vi "fgt get controllers info.vi"(8 "error in (no error)":errorcluster) -> (0 "error out":errorcluster, 3 "Controllers channels info":T1[](array[typedef]))   [LabVIEW 2016, in "fgt_SDK.lvlib"]
doc: "Retrieve information about session controllers. Controllers are MFCS, Flowboard, Link, IPS and Switchboard."
uses:
  fgt_SDK.lvlib
  TypeDefs/fgt_CONTROLLER_INFO.ctl
  TypeDefs/fgt_INSTRUMENT_TYPE.ctl
  dlls/fgt_SDK_32.dll
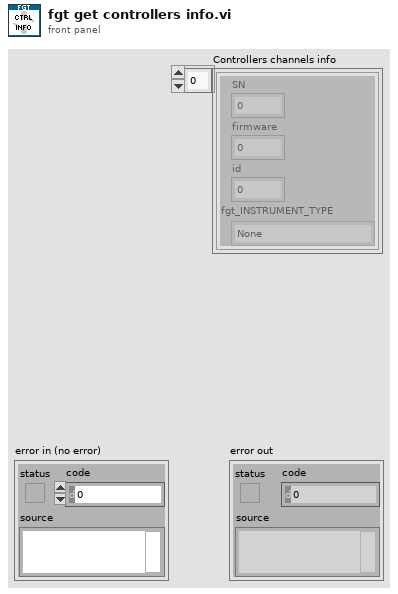
[diagram p1: front panel]
types:
  T1 = typedef "fgt_SDK.lvlib/fgt_CONTROLLER_INFO.ctl" = cluster{"SN":u16, "firmware":u16, "id":u32, "fgt_INSTRUMENT_TYPE":T2}
  T2 = typedef "fgt_SDK.lvlib/fgt_INSTRUMENT_TYPE.ctl" = enum32{"None", "MFCS", "MFCS_EZ", "FRP", "LineUP", "IPS"}
  T3 = typedef "fgt_SDK.lvlib/fgt_STATUS_INFO.ctl" = cluster{"InstrType":T2, "instrSN":u16, "errorCode":u8, "infoCode":u8, "detail":string}
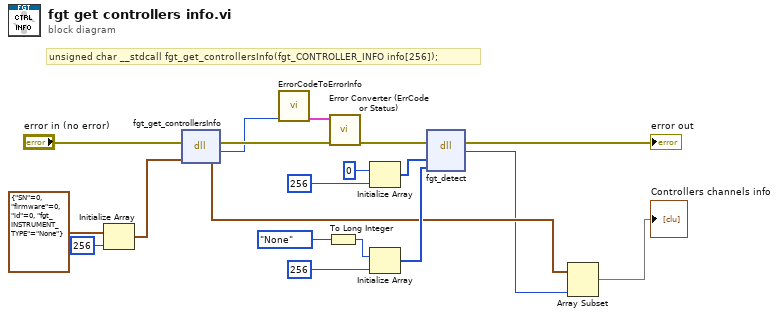
[diagram p0: block diagram]
diagram:
  # "unsigned char __stdcall fgt_get_controllersInfo(fgt_CONTROLLER_INFO info[256]);"
  n1 = Initialize Array(T1 {"SN"=0, "firmware"=0, "id"=0, "fgt_INSTRUMENT_TYPE"=enum."None"} ("fgt_CONTROLLER_INFO"), 256 ("dimension size")) -> (w13:T1[])
  n2 = dll-call lib="C:/projects/SDK/fgt-sdk-labview/dlls/fgt_SDK_*.*" fn="fgt_get_controllersInfo"(error in="error in (no error)", "info"=w13) -> (error out=w18:errorcluster, "return type"=w17:u8, "info"=w3:T1[])  [unwired: 2 in, 1 out]
  n3 = call "ErrorCodeToErrorInfo.vi"("return type"=w17) -> ("StatusInfo"=w16:T3)  [unwired: 10 in]
  n4 = To Long Integer(number=fgt_INSTRUMENT_TYPE."None" ("fgt_INSTRUMENT_TYPE")) -> (32bit integer=w7:i32)
  n5 = call "Error Converter (ErrCode or Status).vi"("error in (no error)"=w18, "StatusInfo"=w16) -> ("error out"=w5:errorcluster)  [unwired: 9 in]
  n6 = Initialize Array(u16 0 ("element"), 256 ("dimension size")) -> (w6:u16[])
  n7 = Initialize Array(w7, 256 ("dimension size")) -> (w9:i32[])
  n8 = dll-call lib="C:/projects/SDK/fgt-sdk-labview/dlls/fgt_SDK_*.*" fn="fgt_detect"(error in=w5, "SN"=w6, "type"=w9) -> (error out=→"error out":errorcluster, "return type"=w1:u8)  [unwired: 4 in, 1 out]
  n9 = Array Subset(array=w3, length=w1) -> (→"Controllers channels info":T1[])  [unwired: 1 in]
